vi "WriteDblData.vi"(8 "Error In":errorcluster caption="エラー入力", 9 "数値":dbl, 10 "データ":T2, 11 "refnum":T1) -> (0 "Error Out":errorcluster caption="エラー出力", 3 "refnum out":T1 caption="refnum出力")   [LabVIEW 2014]
doc: "iniファイルへDBLデータを書込みます。"
uses:
  <vilib>/Utility/config.llb/NI_LVConfig.lvlib
  <vilib>/Utility/config.llb/Write Key (Double).vi
  <vilib>/Utility/config.llb/Config Data RefNum.ctl
panel:
  # "■IniファイルへDBLデータを書き込む"
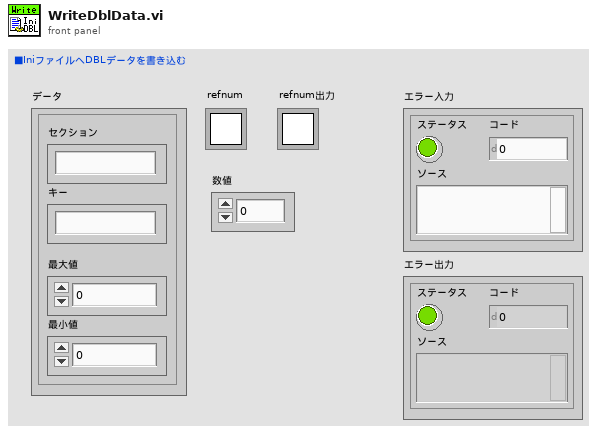
[diagram p1: front panel]
types:
  T1 = typedef "NI_LVConfig.lvlib/Config Data RefNum.ctl" = refnum<k1>
  T2 = cluster{"セクション":string, "キー":string, "最大値":dbl, "最小値":dbl}
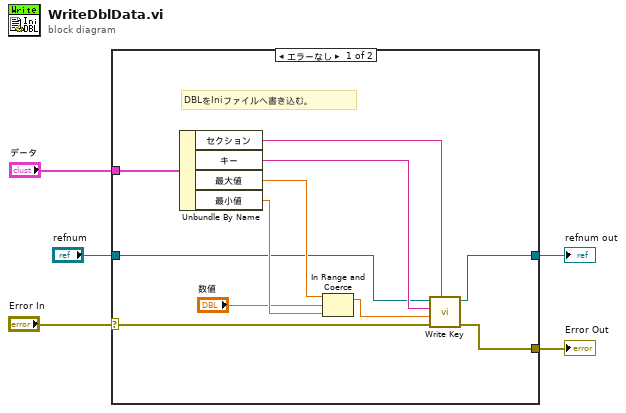
[diagram p0: block diagram]
diagram:
  n1 = case shown="エラーなし" "Error In" {
    selector: "Error In" -> [w13 w18]
    tunnel: [w12 w18] -> w5
    tunnel: "データ" -> [w16 _]
    tunnel: [w6 w17] -> w2
    tunnel: "refnum" -> [w7 w17]
    frame No Error {
      # "DBLをIniファイルへ書き込む。"
      n2 = Unbundle By Name(w16) -> ("セクション"=w15:string, "キー"=w14:string, "最大値"=w11:dbl, "最小値"=w10:dbl)
      n3 = In Range and Coerce(upper limit=w11, x="数値", lower limit=w10) -> (coerced(x)=w8:dbl)  [unwired: 1 out]
      n4 = call-poly <vilib>:"Write Key.vi"("section"=w15, "error in (no error)"=w13, "value"=w8, "key"=w14, "refnum"=w7) -> ("error out"=w12:errorcluster, "refnum out"=w6:T1)  [unwired: 4 in, 1 out]
    }
    frame Error {
    }
  }
  "Error Out" <- w5
  "refnum out" <- w2
